vi "Get Simple Channel Name.vi"(11 "channel":refnum<class "TBM channel.lvclass">) -> (3 "channel 2":refnum<class "TBM channel.lvclass">)   [LabVIEW 2013, in "Scan Engine editor node.lvclass"]
uses:
  Scan Engine editor node.lvclass
  <vilib>/NI/Tag Bus Module Framework/channel/TBM channel.lvclass
  <vilib>/NI/Tag Bus/tag/tag descriptor.lvclass/tag descriptor.ctl
  <vilib>/NI/Tag Bus/tag/tag descriptor.lvclass
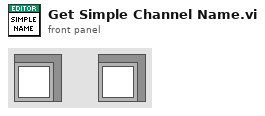
[diagram p1: front panel]
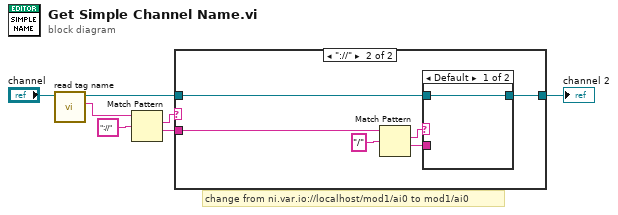
[diagram p0: block diagram]
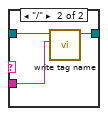
[diagram p3: hidden frame]
diagram:
  # "change from ni.var.io://localhost/mod1/ai0 to mod1/ai0"
  n1 = call <vilib>:"read tag name.vi"("system tag in"="channel") -> ("name"=w6:string, "system tag out"=w7:refnum<class "TBM channel.lvclass">)  [unwired: 8 in, 1 out]
  n2 = Match Pattern(string=w6, regular expression="://") -> (match substring=w4:string, after substring=w3:string)  [unwired: 1 in, 2 out]
  n3 = case shown="\"://\"" w4 {
    tunnel: [w8 w14] -> w1
    tunnel: w7 -> [w8 w13]
    tunnel: w3 -> [_ w12]
    frame Default {
    }
    frame "://" {
      n4 = Match Pattern(string=w12, regular expression="/") -> (match substring=w10:string, after substring=w9:string)  [unwired: 1 in, 2 out]
      n5 = case shown="Default" w10 {
        tunnel: [w15 w18] -> w14
        tunnel: w13 -> [w15 w17]
        tunnel: w9 -> [_ w16]
        frame Default {
        }
        frame "/" {
          n6 = call <vilib>:"write tag name.vi"("name"=w16, "system tag in"=w17) -> ("system tag out"=w18:refnum<class "TBM channel.lvclass">)  [unwired: 8 in, 1 out]
        }
      }
    }
  }
  "channel 2" <- w1
